vi "Pockels-Convert AO sequence from time to samples.vi"(8 "Direction (+Inf)":T1=enum."Toward +Inf", 11 "Duration of AO sequence (us)":dbl format="%#_6f") -> (3 "Number of samples in AO sequence":i32)   [LabVIEW 2013]
uses:
  Typedefs/Rounding type.ctl
  Global Variables/General Globals.vi
panel:
  out "Sampling period (us)":dbl
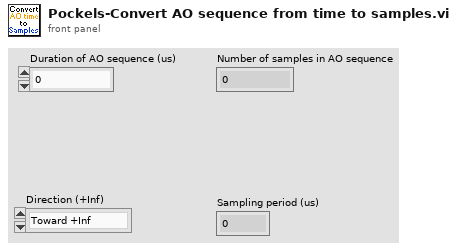
[diagram p1: front panel]
types:
  T1 = typedef "Rounding type.ctl" = enum16{"No rounding", "Toward +Inf", "Toward -Inf"}
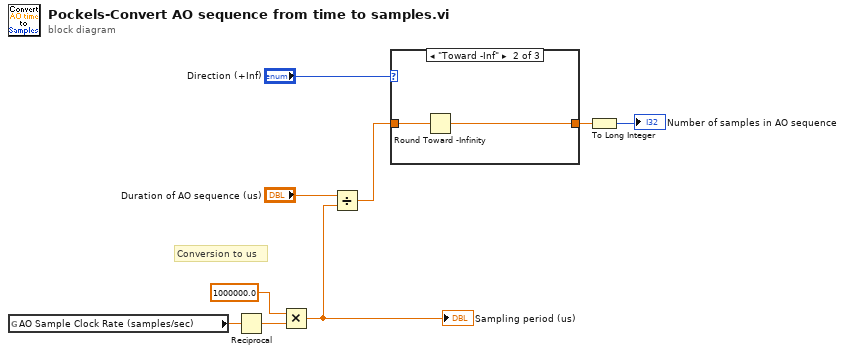
[diagram p0: block diagram]
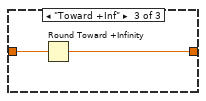
[diagram p3: hidden frame]
diagram:
  # "Conversion to us"
  n1 = global read "General Globals.vi" "AO Sample Clock Rate (samples/sec)"() -> (w2:dbl)
  n2 = Reciprocal(x=w2) -> (1/x=w8:dbl)
  n3 = Multiply(x=1000000.0 ("y"), y=w8) -> (x*y=w7:dbl)
  "Sampling period (us)" <- w7
  n4 = Divide(x="Duration of AO sequence (us)", y=w7) -> (x/y=w1:dbl)
  n5 = case shown="\"Toward -Inf\"" "Direction (+Inf)" {
    tunnel: w1 -> [w10 w12 w14]
    tunnel: [w10 w11 w13] -> w9
    frame "No rounding", Default {
    }
    frame "Toward -Inf" {
      n6 = Round Toward -Infinity(1:w12) -> (0:w11:dbl)
    }
    frame "Toward +Inf" {
      n7 = Round Toward +Infinity(x=w14) -> (ceil(x): smallest int >= x=w13:dbl)
    }
  }
  n8 = To Long Integer(number=w9) -> (32bit integer=→"Number of samples in AO sequence":i32)
